vi "Motors Status Bk.vi"(2 "error in":errorcluster, 3 "VISA in":refnum<visa-resource-name>) -> (0 "error out":errorcluster, 1 "VISA out":refnum<visa-resource-name>)   [LabVIEW 2010]
panel:
  out "Jogger Fast Speed (mm/s)":string
  out "Jogger Speed (mm/s)":string
  out "Jogger buffer":string
  out "OA":string
  out "OA buffer":string
  out "OS":string
  out "OS buffer":string
  in  "Axis":i32
  out "CO":string
  out "CO buffer":string
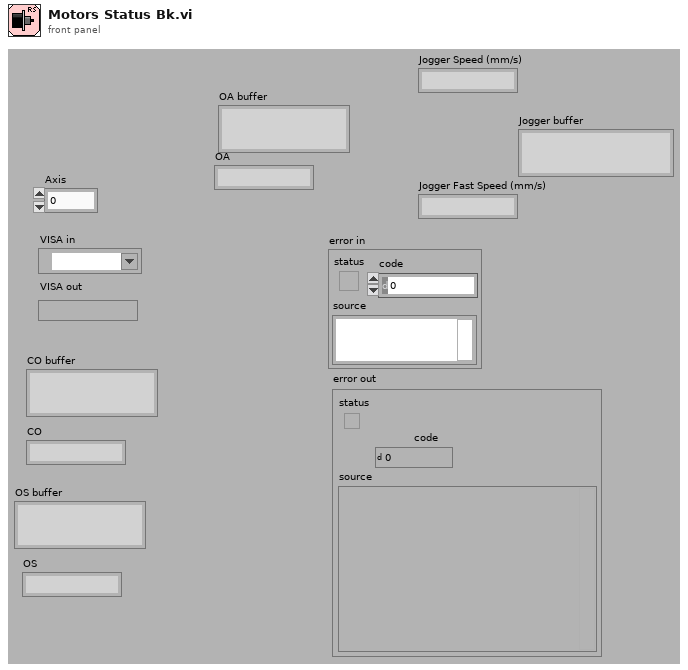
[diagram p1: front panel]
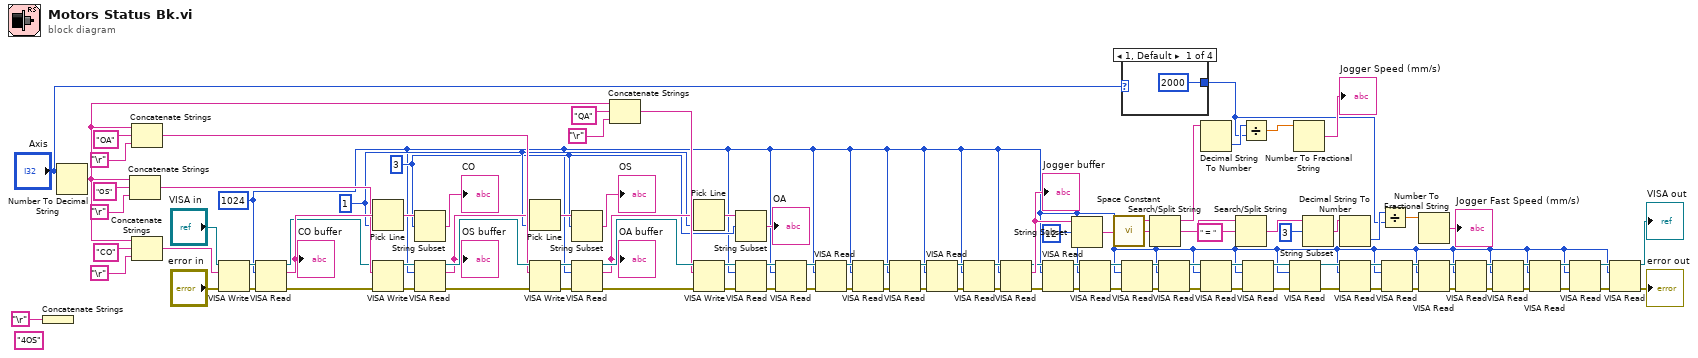
[diagram p0: block diagram]
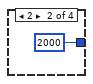
[diagram p2: hidden frame]
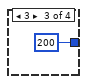
[diagram p3: hidden frame]
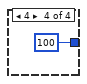
[diagram p4: hidden frame]
diagram:
  (unwired) "4OS" ("Initial command 1")
  w69 = 3 ("offset (0)")
  w71 = 1 ("line index")
  w15 = u32 1024 ("byte count")
  n1 = Concatenate Strings("\r") -> ()  [unwired: 1 out]
  n2 = Number To Decimal String(number="Axis") -> (decimal integer string=w67:string)  [unwired: 1 in]
  n3 = Concatenate Strings(w67, "OS" ("Initial command 1"), "\r") -> (w82:string)
  n4 = Concatenate Strings(w67, "OA" ("Initial command 1"), "\r") -> (w81:string)
  n5 = Concatenate Strings(w67, "CO" ("Initial command 1"), "\r") -> (w104:string)
  n6 = VISA Write(VISA resource name="VISA in", write buffer=w104, error in (no error)="error in") -> (VISA resource name out=w102:refnum<visa-resource-name>, error out=w103:errorcluster)  [unwired: 1 out]
  n7 = VISA Read(VISA resource name=w102, byte count=w15, error in (no error)=w103) -> (VISA resource name out=w79:refnum<visa-resource-name>, read buffer=w99:string, error out=w78:errorcluster)  [unwired: 1 out]
  "CO buffer" <- w99
  n8 = Pick Line(multi-line string=w99, line index=w71) -> (output string=w98:string)  [unwired: 1 in]
  n9 = VISA Write(VISA resource name=w79, write buffer=w82, error in (no error)=w78) -> (VISA resource name out=w96:refnum<visa-resource-name>, error out=w95:errorcluster)  [unwired: 1 out]
  n10 = String Subset(string=w98, offset (0)=w69) -> (substring=→"CO":string)  [unwired: 1 in]
  n11 = VISA Read(VISA resource name=w96, byte count=w15, error in (no error)=w95) -> (VISA resource name out=w94:refnum<visa-resource-name>, read buffer=w76:string, error out=w93:errorcluster)  [unwired: 1 out]
  "OS buffer" <- w76
  n12 = Pick Line(multi-line string=w76, line index=w71) -> (output string=w75:string)  [unwired: 1 in]
  n13 = VISA Write(VISA resource name=w94, write buffer=w81, error in (no error)=w93) -> (VISA resource name out=w92:refnum<visa-resource-name>, error out=w91:errorcluster)  [unwired: 1 out]
  n14 = String Subset(string=w75, offset (0)=w69) -> (substring=→"OS":string)  [unwired: 1 in]
  n15 = VISA Read(VISA resource name=w92, byte count=w15, error in (no error)=w91) -> (VISA resource name out=w88:refnum<visa-resource-name>, read buffer=w72:string, error out=w87:errorcluster)  [unwired: 1 out]
  "OA buffer" <- w72
  n16 = Concatenate Strings(w67, "QA" ("Initial command 1"), "\r") -> (w80:string)
  n17 = Pick Line(multi-line string=w72, line index=w71) -> (output string=w70:string)  [unwired: 1 in]
  n18 = VISA Write(VISA resource name=w88, write buffer=w80, error in (no error)=w87) -> (VISA resource name out=w89:refnum<visa-resource-name>, error out=w90:errorcluster)  [unwired: 1 out]
  n19 = String Subset(string=w70, offset (0)=w69) -> (substring=→"OA":string)  [unwired: 1 in]
  n20 = VISA Read(VISA resource name=w89, byte count=w15, error in (no error)=w90) -> (VISA resource name out=w65:refnum<visa-resource-name>, error out=w64:errorcluster)  [unwired: 2 out]
  n21 = VISA Read(VISA resource name=w65, byte count=w15, error in (no error)=w64) -> (VISA resource name out=w61:refnum<visa-resource-name>, error out=w60:errorcluster)  [unwired: 2 out]
  n22 = VISA Read(VISA resource name=w61, byte count=w15, error in (no error)=w60) -> (VISA resource name out=w62:refnum<visa-resource-name>, error out=w63:errorcluster)  [unwired: 2 out]
  n23 = VISA Read(VISA resource name=w62, byte count=w15, error in (no error)=w63) -> (VISA resource name out=w59:refnum<visa-resource-name>, error out=w58:errorcluster)  [unwired: 2 out]
  n24 = VISA Read(VISA resource name=w59, byte count=w15, error in (no error)=w58) -> (VISA resource name out=w57:refnum<visa-resource-name>, error out=w56:errorcluster)  [unwired: 2 out]
  n25 = VISA Read(VISA resource name=w57, byte count=w15, error in (no error)=w56) -> (VISA resource name out=w55:refnum<visa-resource-name>, error out=w53:errorcluster)  [unwired: 2 out]
  n26 = VISA Read(VISA resource name=w55, byte count=w15, error in (no error)=w53) -> (VISA resource name out=w54:refnum<visa-resource-name>, error out=w52:errorcluster)  [unwired: 2 out]
  n27 = VISA Read(VISA resource name=w54, byte count=w15, error in (no error)=w52) -> (VISA resource name out=w29:refnum<visa-resource-name>, read buffer=w51:string, error out=w14:errorcluster)  [unwired: 1 out]
  "Jogger buffer" <- w51
  n28 = VISA Read(VISA resource name=w29, byte count=w15, error in (no error)=w14) -> (VISA resource name out=w32:refnum<visa-resource-name>, error out=w33:errorcluster)  [unwired: 2 out]
  n29 = String Subset(string=w51, offset (0)=12) -> (substring=w49:string)  [unwired: 1 in]
  n30 = VISA Read(VISA resource name=w32, byte count=w15, error in (no error)=w33) -> (VISA resource name out=w28:refnum<visa-resource-name>, error out=w13:errorcluster)  [unwired: 2 out]
  n31 = call <vilib>:"Space Constant.vi"() -> ("String"=w48:string)
  n32 = case shown="1, Default" "Axis" {
    tunnel: [2000 2000 200 100] -> w36
    frame 1, Default {
    }
    frame 2 {
    }
    frame 3 {
    }
    frame 4 {
    }
  }
  n33 = VISA Read(VISA resource name=w28, byte count=w15, error in (no error)=w13) -> (VISA resource name out=w27:refnum<visa-resource-name>, error out=w12:errorcluster)  [unwired: 2 out]
  n34 = Search/Split String(string=w49, search string/char (-)=w48) -> (substring before match=w43:string, match + rest of string=w44:string)  [unwired: 1 in, 1 out]
  n35 = VISA Read(VISA resource name=w27, byte count=w15, error in (no error)=w12) -> (VISA resource name out=w26:refnum<visa-resource-name>, error out=w11:errorcluster)  [unwired: 2 out]
  n36 = Decimal String To Number(string=w43) -> (number=w41:i32)  [unwired: 2 in, 1 out]
  n37 = VISA Read(VISA resource name=w26, byte count=w15, error in (no error)=w11) -> (VISA resource name out=w25:refnum<visa-resource-name>, error out=w10:errorcluster)  [unwired: 2 out]
  n38 = Search/Split String(string=w44, search string/char (-)=" = ") -> (match + rest of string=w46:string)  [unwired: 1 in, 2 out]
  n39 = Divide(x=w41, y=w36) -> (x/y=w38:dbl)
  n40 = VISA Read(VISA resource name=w25, byte count=w15, error in (no error)=w10) -> (VISA resource name out=w24:refnum<visa-resource-name>, error out=w9:errorcluster)  [unwired: 2 out]
  n41 = VISA Read(VISA resource name=w24, byte count=w15, error in (no error)=w9) -> (VISA resource name out=w23:refnum<visa-resource-name>, error out=w8:errorcluster)  [unwired: 2 out]
  n42 = Number To Fractional String(number=w38) -> (F-format string=→"Jogger Speed (mm/s)":string)  [unwired: 3 in]
  n43 = String Subset(string=w46, offset (0)=3) -> (substring=w42:string)  [unwired: 1 in]
  n44 = Decimal String To Number(string=w42) -> (number=w40:i32)  [unwired: 2 in, 1 out]
  n45 = VISA Read(VISA resource name=w23, byte count=w15, error in (no error)=w8) -> (VISA resource name out=w22:refnum<visa-resource-name>, error out=w7:errorcluster)  [unwired: 2 out]
  n46 = Divide(x=w40, y=w36) -> (x/y=w35:dbl)
  n47 = VISA Read(VISA resource name=w22, byte count=w15, error in (no error)=w7) -> (VISA resource name out=w21:refnum<visa-resource-name>, error out=w6:errorcluster)  [unwired: 2 out]
  n48 = Number To Fractional String(number=w35) -> (F-format string=→"Jogger Fast Speed (mm/s)":string)  [unwired: 3 in]
  n49 = VISA Read(VISA resource name=w21, byte count=w15, error in (no error)=w6) -> (VISA resource name out=w20:refnum<visa-resource-name>, error out=w5:errorcluster)  [unwired: 2 out]
  n50 = VISA Read(VISA resource name=w20, byte count=w15, error in (no error)=w5) -> (VISA resource name out=w30:refnum<visa-resource-name>, error out=w31:errorcluster)  [unwired: 2 out]
  n51 = VISA Read(VISA resource name=w30, byte count=w15, error in (no error)=w31) -> (VISA resource name out=w19:refnum<visa-resource-name>, error out=w4:errorcluster)  [unwired: 2 out]
  n52 = VISA Read(VISA resource name=w19, byte count=w15, error in (no error)=w4) -> (VISA resource name out=w18:refnum<visa-resource-name>, error out=w3:errorcluster)  [unwired: 2 out]
  n53 = VISA Read(VISA resource name=w18, byte count=w15, error in (no error)=w3) -> (VISA resource name out=w17:refnum<visa-resource-name>, error out=w2:errorcluster)  [unwired: 2 out]
  n54 = VISA Read(VISA resource name=w17, byte count=w15, error in (no error)=w2) -> (VISA resource name out=→"VISA out":refnum<visa-resource-name>, error out=→"error out":errorcluster)  [unwired: 2 out]
